vi "One Shot Single Tone - no AO.vi"() -> ()   [LabVIEW 2021]
doc: "This VI generates and acquires data for a single-shot acquisition and performs gain and total harmonic distortion (THD) measurements on the acquired response channel. You can specify the initial settling time of the device under test, the integration time to use for the measurement, and the frequency range of interest. \n\nThe graphical outputs display the time record of the acquired response and the magnitude spectrum versus frequency, respectively. You can also investigate the contribution of each harmonic component to the THD.\n\nRequirements:\nLabVIEW Full Development System\nSound and Vibration Toolkit\n\nInstructions:\n1. Connect DUT to DAQmx hardware.\n2. Specify connected output channel and input channel (response).\n3. Use SVL Measure Propagation Delay (DAQmx) VI to measure device propagation delay [samples].\n4. Run the VI.\n\nDetails:\nThis VI measures the gain and total harmonic distortion (THD) of a device under test (DUT). It generates a single-tone stimulus to excite the DUT. The gain is the ratio of output to input amplitudes. THD quantifies the level of non-linear harmonics produced from excitation at a single frequency. THD is defined as the ratio of the RMS sum of the harmonic levels to the level of the fundamental frequency. \n\nRefer to the wiring diagram to physically connect the DSA or DAQ device to the DUT. This example uses one analog input channel and one analog output channel. \n\nThe wiring diagram assumes that you use the default channel settings. If you change the channel settings in the VI front panel you should adjust the physical connections appropriately.\n\nNI strongly recommends that you take precautions to limit the effects of out-of-band aliasing in your frequency domain measurements. DSA devices use transparent digital and analog hardware filtering to eliminate aliased input and output frequencies. Multifunction DAQ devices are more susceptible to the effects of aliased frequencies. If you are using a non-DSA measurement device, we recommend addressing potential aliasing through high sampling rates, built-in analog filters on S Series devices, and/or external analog filters."
uses:
  <vilib>/addons/_XControls/Spectrum with Cursors/Spectrum with Cursors.xctl
  <vilib>/addons/_NISVFA/_Shared subVIs/Data Objects/Data/Data.lvclass
  <vilib>/addons/_XControls/Waveforms with Cursors/Waveforms with Cursors.xctl
  <vilib>/addons/_NISVFA/_Generation/Signal Generation/SV Signal/sv_System Timing Model.ctl
  Program Files/National Instruments/LabVIEW 2021/examples/Sound and Vibration/Audio Measurements/subVIs/sv_AO Channel Configuration.ctl
  Program Files/National Instruments/LabVIEW 2021/examples/Sound and Vibration/Audio Measurements/subVIs/sv_AI Channel Configuration.ctl
  <vilib>/addons/_NISVFA/_Generation/Signal Generation/SV Signal/SV Signal.lvclass/SV Signal.ctl
  <vilib>/addons/_NISVFA/_Shared subVIs/Controls/svc_Window.ctl
  <vilib>/addons/_NISVFA/_Shared subVIs/Data Objects/Data/Data.lvclass/Data.ctl
  <vilib>/addons/_NISVFA/_Generation/Signal Generation/SV Signal/Write Synchronization Pulse Parameters.vi
  <vilib>/addons/_NISVFA/_Generation/Signal Generation/SV Signal/Write Ramp-Up.vi
  <vilib>/addons/_NISVFA/_Generation/Signal Generation/SV Signal/Write Ramp-Down.vi
  <vilib>/addons/_NISVFA/_Generation/Signal Generation/SV Signal/Write Profile.vi
  <vilib>/Analysis/1siggen.llb/Ramp Pattern by Samples.vi
  <vilib>/addons/_NISVFA/_Shared subVIs/Common/SVL Set dB Reference (1 Ch).vi
  <vilib>/addons/Sound and Vibration/svt_Level/SVL AC & DC Level (Time) (1 Ch).vi
  <vilib>/addons/_NISVFA/_Shared subVIs/Data Objects/Y (Complex) (DBL)/SV Convert Complex Spectrum to Data Object.vi
  <vilib>/addons/Sound and Vibration/svt_Single Tone Measurements/SVT Spurious Free Dynamic Range (Frequency) (1 Ch).vi
  <vilib>/DAQmx/read.llb/DAQmx Read.vi
  <vilib>/DAQmx/read.llb/DAQmx Read (Analog 1D Wfm NChan NSamp).vi
  Program Files/National Instruments/LabVIEW 2021/examples/Sound and Vibration/Audio Measurements/subVIs/sv_Modify Channel Names.vi
  Program Files/National Instruments/LabVIEW 2021/examples/Sound and Vibration/Audio Measurements/subVIs/sv_Synchronize DSA AI and AO Tasks.vi
  <vilib>/DAQmx/write.llb/DAQmx Write.vi
  <vilib>/DAQmx/write.llb/DAQmx Write (Analog Wfm 1Chan NSamp).vi
  Program Files/National Instruments/LabVIEW 2021/examples/Sound and Vibration/Audio Measurements/subVIs/sv_Synchronization Gatekeeper.vi
  Program Files/National Instruments/LabVIEW 2021/examples/Sound and Vibration/Audio Measurements/subVIs/sv_Synchronize Acquisition and Generation.vi
  Program Files/National Instruments/LabVIEW 2021/examples/Sound and Vibration/Audio Measurements/subVIs/sv_Prepare Acquired Waveforms for Parsing.vi
  <vilib>/addons/_NISVFA/_Shared subVIs/Common/SVL Set dB Reference (variant).vi
  <vilib>/addons/_NISVFA/_Shared subVIs/Common/svc_Get SV Channel Info.vi
  <vilib>/Analysis/baseanly.llb/Mean.vi
  <vilib>/Analysis/baseanly.llb/Mean (DBL).vi
  <vilib>/addons/_NISVFA/_Shared subVIs/Windowing/svfa_Scaled Time Domain Window (Array).vi
  <vilib>/addons/_NISVFA/_Shared subVIs/Common/sv_Get NI Property Name String.vi
  <vilib>/addons/_NISVFA/_Shared subVIs/Data Objects/Data/Write Data Attributes.vi
  <vilib>/addons/_NISVFA/_Spectrum Processing/SVFA Get Spectrum Subset.vi
  <vilib>/addons/_NISVFA/_Spectrum Processing/SVFA Get Spectrum Subset (Complex) (1 Ch).vi
  <vilib>/addons/_NISVFA/_Shared subVIs/Common/svc_Window Parameters.vi
  <vilib>/addons/_NISVFA/_Shared subVIs/Common/svc_Extract Single Tone Information (complex).vi
  <vilib>/addons/_NISVFA/_Shared subVIs/Common/svc_Check Frequency Range in Spectrum.vi
  <vilib>/addons/_NISVFA/_Spectrum Processing/SVFA Unit Conversion.vi
  <vilib>/addons/_NISVFA/_Spectrum Processing/SVFA Unit Conversion (Complex) (1 Ch).vi
  <vilib>/addons/_NISVFA/_Spectrum Processing/SVFA Spectrum Peak Search.vi
  <vilib>/addons/_NISVFA/_Spectrum Processing/SVFA Spectrum Peak Search (1 Ch).vi
  <vilib>/addons/_NISVFA/_Shared subVIs/Common/svc_Spectrum Units.vi
  Program Files/National Instruments/LabVIEW 2021/examples/Sound and Vibration/Audio Measurements/subVIs/sv_Synchronization Keymaster.vi
  <vilib>/Utility/error.llb/Clear Errors.vi
  Program Files/National Instruments/LabVIEW 2021/examples/Sound and Vibration/Audio Measurements/subVIs/sv_Get Reference Clock.vi
  Program Files/National Instruments/LabVIEW 2021/examples/Sound and Vibration/Audio Measurements/subVIs/sv_Synchronization Keymaster_GO.vi
  <extravilib>/ChannelInstances/Tag-c(ref(UserDefinedRefnumTag),t'Rendezvous RefNum')/Read.vi
  Program Files/National Instruments/LabVIEW 2021/examples/Sound and Vibration/Audio Measurements/subVIs/sv_Timing for Stimulus Response Tasks.vi
  <vilib>/addons/_NISVFA/_Generation/Signal Generation/SV Signal/Read Total Samples.vi
  <vilib>/addons/_NISVFA/_Generation/Signal Generation/SV Signal/Write Leading Synchronization Pulse Enable.vi
  Program Files/National Instruments/LabVIEW 2021/examples/Sound and Vibration/Audio Measurements/subVIs/sv_Align Waveforms by Leading Sync Pulse.vi
  <vilib>/addons/_NISVFA/_Generation/Signal Generation/SV Signal/Read Synchronization Pulse Waveform.vi
  <vilib>/addons/_NISVFA/_Shared subVIs/Common/svc_Check for Waveform Parameter Continuity (N Ch).vi
  Program Files/National Instruments/LabVIEW 2021/examples/Sound and Vibration/Audio Measurements/subVIs/sv_Append Virtual Reference.vi
  <vilib>/addons/_NISVFA/_Shared subVIs/Common/svc_Unit Label to Engineering Units.vi
  <vilib>/addons/_NISVFA/_Shared subVIs/Common/svc_Engineering Units to Unit Label.vi
  <vilib>/addons/_NISVFA/_Spectrum Processing/subVIs/svfa_Spectrum Info Window to windowTd Type Def.vi
  <vilib>/Analysis/4window.llb/Force Window.vi
  <vilib>/Analysis/4window.llb/Force Window (DBL).vi
  <vilib>/Analysis/4window.llb/Exponential Window.vi
  <vilib>/Analysis/4window.llb/Exponential Window (DBL).vi
  <vilib>/addons/_NISVFA/_Shared subVIs/Data Objects/Data/Read Data Attributes.vi
  <vilib>/addons/_NISVFA/_Shared subVIs/Common/svc_Build Unit Label for Frequency Range.vi
  <vilib>/addons/_NISVFA/_Spectrum Processing/SVFA Get Tone Amplitude and Phase (1 Ch).vi
  <vilib>/addons/_NISVFA/_Spectrum Processing/subVIs/svfa_Compute Complex Spectrum for Export.vi
  <vilib>/addons/_NISVFA/_Shared subVIs/Common/svc_Check Frequency Range in Bandwidth.vi
  <vilib>/addons/_NISVFA/_Shared subVIs/Common/svc_Convert Start and Stop to Start Index and Length.vi
  <vilib>/addons/_NISVFA/_Shared subVIs/Common/svc_Log View for Spectrum (1Ch).vi
  <vilib>/addons/_NISVFA/_Spectrum Processing/SVFA Unit Conversion (1 Ch).vi
  <vilib>/addons/_NISVFA/_Shared subVIs/Common/svc_Complex Datatype Defaults.vi
  <vilib>/addons/_NISVFA/_Spectrum Processing/subVIs/svfa_Spectrum Peak Search.vi
  <vilib>/addons/_NISVFA/_Shared subVIs/Common/svc_Format Value (DBL).vi
  <vilib>/addons/_NISVFA/_Shared subVIs/Common/svc_Get Weighting Enum and Labels.vi
  <vilib>/addons/_NISVFA/_Shared subVIs/Common/svc_Surround NonAlpha String with Parentheses.vi
  <vilib>/dlg_ctls.llb/Space Constant.vi
  <extravilib>/ChannelInstances/Tag-c(ref(UserDefinedRefnumTag),t'Rendezvous RefNum')/Write.vi
  <extravilib>/ChannelInstances/Tag-c(ref(UserDefinedRefnumTag),t'Rendezvous RefNum')/Read With Abort.vi
  <vilib>/addons/_NISVFA/_Generation/Signal Generation/SV Signal/Calculate Number of Remaining Samples.vi
  Program Files/National Instruments/LabVIEW 2021/examples/Sound and Vibration/Audio Measurements/subVIs/sv_Measure Delay for Active and Idle Channels.vi
  <vilib>/addons/_NISVFA/_Generation/Signal Generation/SV Signal/Read Leading Synchronization Pulse Enable.vi
  <vilib>/addons/_NISVFA/_Generation/Signal Generation/SV Signal/Read Trailing Synchronization Pulse Enable.vi
  <vilib>/addons/_NISVFA/_Shared subVIs/Common/svc_Check for Waveform Parameter Continuity (no state).vi
  <vilib>/addons/_NISVFA/_Spectrum Processing/subVIs/svfa_Window Frequency Response.vi
  <vilib>/addons/_NISVFA/_Spectrum Processing/subVIs/svfa_Window Frequency Response (double array).vi
  <vilib>/Analysis/baseanly.llb/Dot Product.vi
  <vilib>/Analysis/baseanly.llb/Complex Dot Product.vi
  <vilib>/addons/_NISVFA/_Shared subVIs/Common/svc_Unwrap Phase.vi
  <vilib>/addons/_NISVFA/_Shared subVIs/Common/svc_Convert Spectrum Array to dB.vi
  <vilib>/addons/_NISVFA/_Spectrum Processing/subVIs/svfa_Conversion Utility (spectrum info).vi
  <vilib>/addons/_NISVFA/_Spectrum Processing/subVIs/svfa_Peak Rough Search Indices.vi
  <vilib>/addons/_NISVFA/_Shared subVIs/Common/svc_Unit Label Lexical Class.vi
  <extravilib>/ChannelInstances/Tag-c(ref(UserDefinedRefnumTag),t'Rendezvous RefNum')/Write With Abort.vi
  <vilib>/addons/Sound and Vibration/svt_Calibration/SV Measure Delay and Polarity and Coherence (Nx1).vi
  Program Files/National Instruments/LabVIEW 2021/examples/Sound and Vibration/Audio Measurements/subVIs/sv_Assign Delay to Idle Channels.vi
  <vilib>/addons/_NISVFA/_Spectrum Processing/subVIs/svfa_Rect Window Frequency Response.vi
  <vilib>/addons/_NISVFA/_Spectrum Processing/subVIs/svfa_Cosine Window Coefficients.vi
  <vilib>/addons/_NISVFA/_Spectrum Processing/subVIs/svfa_Peak to RMS to Peak2Peak.vi
  <vilib>/addons/_NISVFA/_Spectrum Processing/subVIs/svfa_Mag to Mag2.vi
  <vilib>/addons/_NISVFA/_Spectrum Processing/subVIs/svfa_Linear to dB.vi
  <vilib>/addons/_NISVFA/_Spectrum Processing/subVIs/svfa_dBrefA to dBrefB.vi
  <vilib>/addons/_NISVFA/_Spectrum Processing/subVIs/svfa_Spectrum to Spectral Density.vi
  <vilib>/addons/Sound and Vibration/svt_Calibration/SV Measure Delay and Polarity and Coherence.vi
  <vilib>/Analysis/_algsub.llb/Vector Norm.vi
  <vilib>/Analysis/_algsub.llb/Real Vector Norm.vi
  <vilib>/addons/_NISVFA/_Shared subVIs/Common/SV Get Data Subset.vi
  <vilib>/addons/_NISVFA/_Shared subVIs/Common/svc_Get Array Subset (Index).vi
  <vilib>/addons/_NISVFA/_Shared subVIs/Common/svc_Coerce Index and Length.vi
  <vilib>/addons/_NISVFA/_Shared subVIs/Common/svc_Conditional Merge Error.vi
  <vilib>/addons/_NISVFA/_Generation/Signal Generation/SV Sinusoid/SV Sinusoid.lvclass
  C:/Program Files/National Instruments/LabVIEW 2021/vi.lib/addons/_NISVFA/_Generation/Signal Generation/SV Signal/SV Signal.lvclass
  C:/Program Files/National Instruments/LabVIEW 2021/vi.lib/addons/_NISVFA/_Generation/Signal Generation/SV Function/SV Function.lvclass
  <vilib>/addons/_NISVFA/_Shared subVIs/Data Objects/Y (Complex) (DBL)/Y (Complex) (1 Ch).lvclass
  C:/Program Files/National Instruments/LabVIEW 2021/vi.lib/addons/_NISVFA/_Shared subVIs/Data Objects/Data/Data.lvclass
  <vilib>/addons/_NISVFA/_Generation/Signal Generation/SV Sinusoid/Configure Sine.vi
  <vilib>/addons/_NISVFA/_Generation/Signal Generation/SV Signal/Write System Timing Model.vi
  <vilib>/addons/_NISVFA/_Generation/Signal Generation/SV Signal/Write Transition Profile.vi
  <vilib>/addons/_NISVFA/_Generation/Signal Generation/SV Signal/Write Measurement Duration.vi
  <vilib>/addons/_NISVFA/_Generation/Signal Generation/SV Function/Write Measurement Cycles.vi
  <vilib>/addons/_NISVFA/_Generation/Signal Generation/SV Signal/Write Pre-Measurement Settling Duration.vi
  <vilib>/addons/_NISVFA/_Generation/Signal Generation/SV Function/Write Pre-Measurement Settling Cycles.vi
  <extravilib>/ChannelInstances/Tag-c(ref(UserDefinedRefnumTag),t'Rendezvous RefNum')/Instantiate.vi
  Program Files/National Instruments/LabVIEW 2021/examples/Sound and Vibration/Audio Measurements/subVIs/sv_Configure AI Task.vi
  Program Files/National Instruments/LabVIEW 2021/examples/Sound and Vibration/Audio Measurements/subVIs/sv_Configure AO Task.vi
  <vilib>/addons/_NISVFA/_Generation/Signal Generation/SV Signal/Read Sample Rate.vi
  <vilib>/addons/_NISVFA/_Generation/Signal Generation/SV Signal/Read Generation State.vi
  <vilib>/addons/_NISVFA/_Generation/Signal Generation/SV Signal/Read System Timing Model.vi
  <vilib>/DAQmx/configure/timing.llb/DAQmx Timing.vi
  <vilib>/DAQmx/configure/timing.llb/DAQmx Timing (Sample Clock).vi
  <vilib>/addons/_NISVFA/_Generation/Signal Generation/SV Signal/Write Sample Rate.vi
  <extravilib>/ChannelInstances/Tag-c(ref(UserDefinedRefnumTag),t'Rendezvous RefNum')/EndpointRead.vi
  <vilib>/Utility/rendezvs.llb/Wait at Rendezvous.vi
  <vilib>/DAQmx/configure/task.llb/DAQmx Stop Task.vi
  Program Files/National Instruments/LabVIEW 2021/examples/Sound and Vibration/Audio Measurements/subVIs/sv_Get Bus Type and Product Type.vi
  <vilib>/DAQmx/configure/task.llb/DAQmx Control Task.vi
  <vilib>/Utility/rendezvs.llb/Create Rendezvous.vi
  <extravilib>/ChannelInstances/Tag-c(ref(UserDefinedRefnumTag),t'Rendezvous RefNum')/Endpoint.vi
  <vilib>/addons/Sound and Vibration/svt_DAQmx/subVIs/svl_Get Terminal Name with Device Prefix.vi
  <vilib>/DAQmx/configure/trigger.llb/DAQmx Trigger.vi
  <vilib>/DAQmx/configure/trigger.llb/DAQmx Start Trigger (Digital Edge).vi
  <vilib>/DAQmx/configure/task.llb/DAQmx Start Task.vi
  <vilib>/Utility/rendezvs.llb/Destroy Rendezvous.vi
  <vilib>/DAQmx/miscellaneous.llb/DAQmx Fill In Error Info.vi
  <vilib>/DAQmx/configure/task.llb/DAQmx Clear Task.vi
  <vilib>/addons/_NISVFA/_Shared subVIs/Data Objects/Waveforms (DBL)/Write to Buffer.vi
  <vilib>/addons/_NISVFA/_Shared subVIs/Data Objects/Waveforms (DBL)/Read from Buffer.vi
  <vilib>/addons/_NISVFA/_Shared subVIs/Data Objects/Waveforms (DBL)/SV Read Newest Data.vi
  <vilib>/measure/maresamp.llb/Resample Waveforms (single shot).vi
  <vilib>/measure/maresamp.llb/Resample Waveform (single shot).vi
  <vilib>/addons/_NISVFA/_Shared subVIs/Common/svc_Check dt for Equal Sample Rates.vi
  <vilib>/Waveform/TSOps.llb/Timestamp Subtract.vi
  <vilib>/Analysis/2dsp.llb/CrossCorrelation.vi
  <vilib>/Analysis/2dsp.llb/1D Cross Correlation (DBL).vi
  <vilib>/addons/_NISVFA/_Shared subVIs/Common/svc_Fit Quadratic to Max Three Points in Array.vi
  <vilib>/Utility/error.llb/Error Cluster From Error Code.vi
  <vilib>/addons/_NISVFA/_Shared subVIs/Common/svc_Caller VI Returned in Error Source.vi
  <vilib>/addons/_NISVFA/_Shared subVIs/Common/SV Remove Delays (1,N) from Waveforms (N Ch) (DBL).vi
  <vilib>/addons/_NISVFA/_Shared subVIs/Common/SV Remove Delays from Waveforms.vi
  <vilib>/addons/_NISVFA/_Shared subVIs/Data Objects/Waveforms (DBL)/SV Read Next Measurement Data.vi
  <vilib>/addons/_NISVFA/_Shared subVIs/Common/svc_Get Window Info.vi
  <vilib>/Analysis/0measdsp.llb/Scaled Time Domain Window.vi
  <vilib>/Analysis/0measdsp.llb/Scaled Time Domain Window (DBL).vi
  <vilib>/Analysis/baseanly.llb/Std Deviation and Variance.vi
  <vilib>/addons/Sound and Vibration/svt_Single Tone Measurements/SVT Gain (Time) (1 Ch).vi
  <vilib>/addons/_NISVFA/_Shared subVIs/Data Objects/Y (Complex) (DBL)/Write Y.vi
  <vilib>/addons/_NISVFA/_Shared subVIs/Spectrum Info/sv_Convert Spectrum Info to Variant Attributes.vi
  <vilib>/addons/_NISVFA/_Spectrum Processing/SVFA Extract Multiple Tone Information (Complex) (1 Ch).vi
  <vilib>/addons/Sound and Vibration/svt_Distortion/SVT THD and Harmonic Components (Frequency) (1 Ch).vi
  <vilib>/addons/Sound and Vibration/svt_Distortion/SVT SNR without Harmonics (Frequency) (1 Ch).vi
  <vilib>/addons/Sound and Vibration/svt_Single Tone Measurements/SVT Dynamic Range (Frequency) (1 Ch).vi
  <vilib>/addons/Sound and Vibration/svt_Distortion/subVIs/sv_Check Data Valid (Audio) (1 Ch).vi
  <vilib>/addons/_NISVFA/_Shared subVIs/Common/svc_Convert Frequency to Frequency String.vi
  <vilib>/Analysis/4window.llb/window parameters.vi
  <vilib>/Analysis/4window.llb/Window Properties.vi
  <vilib>/Analysis/4window.llb/Window Properties by Name.vi
  <vilib>/addons/_NISVFA/_Spectrum Processing/subVIs/svfa_Spectrum Peak Tone Search and Estimation (complex).vi
  <vilib>/measure/masignal.llb/Tones and Noise Waveform.vi
  <vilib>/addons/_NISVFA/_Shared subVIs/Common/svc_FFT with Window.vi
  <vilib>/Analysis/1siggen.llb/Square Wave.vi
  <vilib>/addons/_NISVFA/_Spectrum Processing/subVIs/svfa_Three Finger Peak Search.vi
  <vilib>/addons/Sound and Vibration/svt_Distortion/subVIs/sv_Peak View Amplitude (1 Ch).vi
  <vilib>/addons/_NISVFA/_Generation/Signal Generation/SV Signal/SV Signal.lvclass
  <vilib>/addons/Sound and Vibration/svt_Single Tone Measurements/SoundVib_SingleTone.lvlib
  <vilib>/addons/Sound and Vibration/svt_Distortion/SoundVib_Distortion.lvlib
  <vilib>/Analysis/NI_AALBase.lvlib
  Program Files/National Instruments/LabVIEW 2021/examples/Sound and Vibration/SoundVib_Audio Examples.lvlib
panel:
  out "Waveforms with Cursors":waveform(dbl)[](xcontrol)
  out "Spectrum with Cursors":refnum<class "Data.lvclass">(xcontrol)
  in  "Settings":T1(tab)
  in  "AO range":dbl=3.5 format="±  %.3g"
  in  "input channel":tag="Dev1/ai0"
  in  "output channel":tag="Dev1/ao0"
  in  "AI range":dbl=3.0 format="±  %.3g"
  in  "amplitude units":enum16{"V", "dB FS"}(ring)
  in  "full scale (V pk)":dbl=3.16 format="%.3p"
  in  "amplitude":dbl=1.0 format="%.3g"
  in  "frequency (Hz)":dbl=1000.0 min=20.0 max=100000.0 step=1.0 format="%.2f"
  in  "frequency range":T2={"band start (Hz)"=20.0, "band stop (Hz)"=20000.0} {"band stop (Hz)" format="%.2f"; "band start (Hz)" format="%.2f"}
  in  "Rub & Buzz maximum harmonic":i32=20 min=-1 max=1000
  in  "measurement cycles":dbl=20.0 min=1.0
  in  "measurement duration (s)":dbl=0.05 min=0.0 format="%.2p"
  in  "THD maximum harmonic":i32=9 min=-1 max=1000
  in  "settle cycles":dbl=10.0 min=0.0
  in  "settle time (s)":dbl=0.01 min=0.0 format="%.2p"
  in  "ramp down (s)":dbl=0.01 min=0.0 format="%.2p"
  in  "ramp up (s)":dbl=0.02 min=0.0 format="%.2p"
  out "Rub & Buzz distortion (%)":dbl format="%_4g"
  out "THD (dB)":dbl format="%.1f"
  out "gain (dB)":dbl format="%.3f"
  out "fundamental amplitude (V)":dbl format="%_6g"
  out "fundamental frequency (Hz)":dbl format="%_6g"
  out "2X amplitude (V)":dbl format="%_4g"
  out "3X amplitude (V)":dbl format="%_4g"
  out "4X amplitude (V)":dbl format="%_4g"
  out "5X amplitude (V)":dbl format="%_4g"
  out "6X amplitude (V)":dbl format="%_4g"
  out "7X amplitude (V)":dbl format="%_4g"
  out "SNR (dB)":dbl format="%.1f"
  out "THD (%)":dbl format="%_4f"
  out "THD+N (dB)":dbl format="%.1f"
  out "Dynamic Range (dB FS)":dbl format="%.1f"
  out "SFDR (dB)":dbl format="%.1f"
  # "Results"
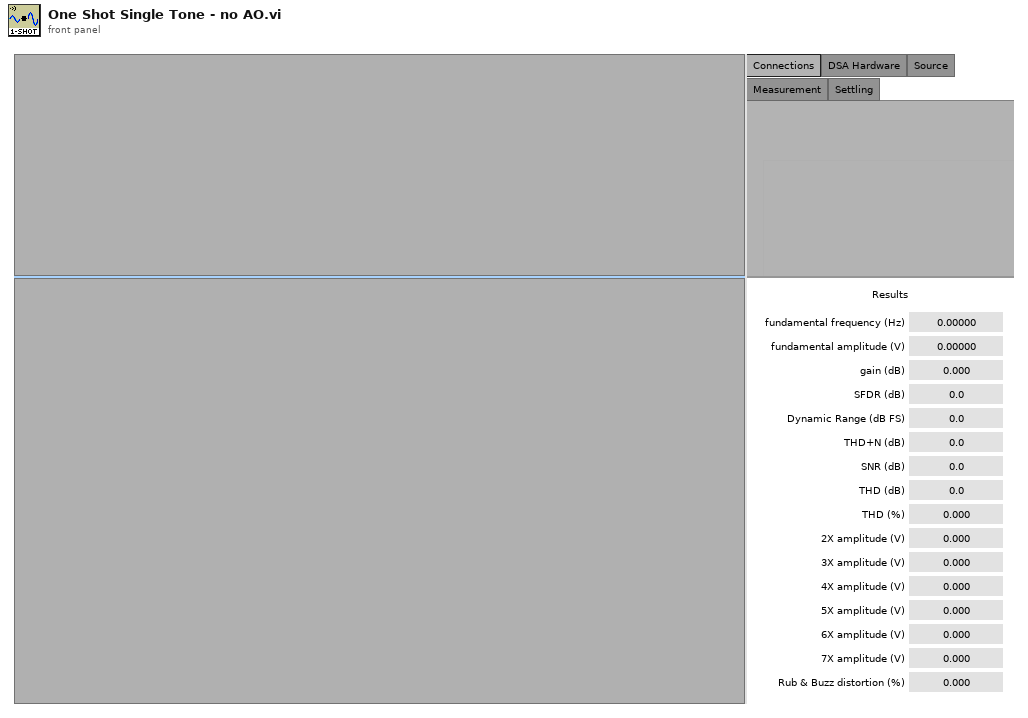
[diagram p1: front panel]
types:
  T1 = enum32{"Connections", "DSA Hardware", "Source", "Measurement", "Settling"}
  T2 = cluster{"band start (Hz)":dbl, "band stop (Hz)":dbl}
  T3 = typedef "SoundVib_Audio Examples.lvlib/sv_AI Channel Configuration.ctl" = cluster{"DAQmx Channel":tag, "Channel Type":u16, "Max":dbl, "Sensitivity":dbl, "Coupling":enum16{"AC", "DC"}, "excitation":enum16{"Off", "Min", "Max"}, "input terminal configuration":i32}
  T4 = typedef "SoundVib_Audio Examples.lvlib/sv_AO Channel Configuration.ctl" = cluster{"DAQmx Channel":tag, "Max":dbl, "output terminal configuration":i32}
  T5 = cluster{"enable leading":bool, "enable trailing":bool, "duration [s]":dbl, "type":enum16{"Noise", "MLS", "Chirp", "Monopulse", "Custom"}, "level":dbl}
  T6 = cluster{"SNR units":enum16{"dB", "linear ratio", "%"}, "detected fundamental amplitude units":enum16{"EU rms", "EU peak", "EU peak-peak"}}
  T7 = cluster{"THD units":enum16{"dB", "linear ratio", "%"}, "harmonic component amplitude units":enum16{"EU rms", "EU peak", "EU peak-peak", "dB ref fund"}, "detected fundamental amplitude units":enum16{"EU rms", "EU peak", "EU peak-peak"}}
  T8 = cluster{"gain units":enum16{"dB", "linear ratio"}, "detected fundamental amplitude units":enum16{"EU rms", "EU peak", "EU peak-peak"}}
  T9 = typedef "SV Signal.lvclass/sv_System Timing Model.ctl" = i64
  T10 = typedef "svc_Window.ctl" = u32
  T11 = typedef "svc_Spectrum Info.ctl" = cluster{"channel name":string, "description":string, "x-axis units":T12, "spectral info":cluster{"spectrum type":T13, "linear/dB":enum16{"linear", "dB"}, "window":u16, "window size":i32, "FFT size":i32}, "engineering units":T14, "custom label":string, "dB reference [EU]":dbl, "peak units":enum16{"rms", "peak", "peak-peak"}, "weighting filter":T15, "spectral density?":bool, "unit label":string, "spectrum skewed?":bool, "complimentary spectrum units":T16}
  T12 = typedef "svc_X-Axis Units.ctl" = u16
  T13 = typedef "svc_Spectrum Type.ctl" = enum16{"FFT Spectrum [complex]", "Amplitude [Magnitude]", "Power [Magnitude^2]", "Cross Spectrum [complex]", "Frequency Response [Complex]"}
  T14 = typedef "svc_Engineering Units Text Ring.ctl" = u16
  T15 = typedef "svc_Weighting Filter Text Ring.ctl" = u16
  T16 = typedef "svc_Complimentary Spectrum Units.ctl" = enum16{"none", "radians", "degrees", "cycles", "imaginary"}
  T17 = cluster{"complex spectrum response":cluster{"f0":dbl, "df":dbl, "complex spectrum":cdb[]}, "spectrum info":T11}
  T18 = cluster{"frequency [Hz]":dbl, "amplitude [EU pk]":dbl, "phase (deg)":dbl}[]
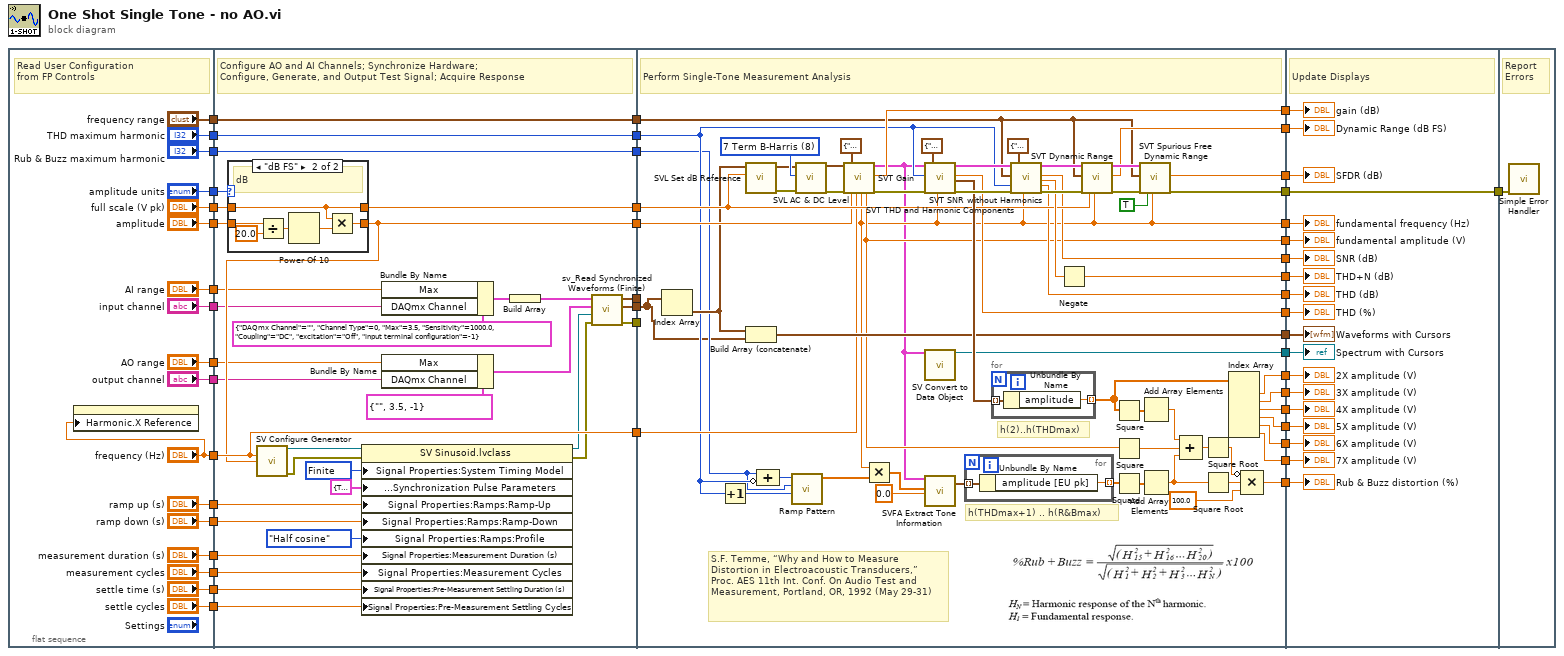
[diagram p0: block diagram]
diagram:
  n1 = flat-sequence {
    tunnel: ["frequency range"] -> w46
    tunnel: ["THD maximum harmonic"] -> w45
    tunnel: ["frequency (Hz)"] -> w44
    tunnel: ["measurement duration (s)"] -> w43
    tunnel: ["measurement cycles"] -> w42
    tunnel: ["settle time (s)"] -> w41
    tunnel: ["settle cycles"] -> w40
    tunnel: ["output channel"] -> w39
    tunnel: ["input channel"] -> w38
    tunnel: ["AI range"] -> w37
    tunnel: ["AO range"] -> w36
    tunnel: ["full scale (V pk)"] -> w35
    tunnel: ["ramp down (s)"] -> w34
    tunnel: ["ramp up (s)"] -> w33
    tunnel: ["amplitude"] -> w32
    tunnel: ["amplitude units"] -> w31
    tunnel: ["Rub & Buzz maximum harmonic"] -> w30
    tunnel: w46 -> [w97]
    tunnel: w45 -> [w87]
    tunnel: w44 -> [w81]
    tunnel: w43 -> [w92]
    tunnel: w42 -> [w91]
    tunnel: w41 -> [w90]
    tunnel: w40 -> [w89]
    tunnel: w39 -> [w64]
    tunnel: w38 -> [w66]
    tunnel: w37 -> [w67]
    tunnel: w36 -> [w65]
    tunnel: w35 -> [w94]
    tunnel: w34 -> [w82]
    tunnel: w33 -> [w83]
    tunnel: w32 -> [w93]
    tunnel: w31 -> [w86]
    tunnel: w30 -> [w85]
    tunnel: [w97] -> w9
    tunnel: [w88] -> w8
    tunnel: [w87] -> w7
    tunnel: [w76] -> w6
    tunnel: [w81] -> w5
    tunnel: [w85] -> w4
    tunnel: [w79] -> w3
    tunnel: [w78] -> w2
    tunnel: [w77] -> w1
    tunnel: [w133] -> w29
    tunnel: [w132] -> w28
    tunnel: [w131] -> w27
    tunnel: [w130] -> w26
    tunnel: [w129] -> w25
    tunnel: [w128] -> w24
    tunnel: [w127] -> w23
    tunnel: [w107] -> w22
    tunnel: [w126] -> w21
    tunnel: [w125] -> w20
    tunnel: [w124] -> w19
    tunnel: [w123] -> w18
    tunnel: [w122] -> w17
    tunnel: [w121] -> w16
    tunnel: [w120] -> w15
    tunnel: [w119] -> w14
    tunnel: [w118] -> w13
    tunnel: [w117] -> w12
    tunnel: [w116] -> w11
    tunnel: w9 -> [w109]
    tunnel: w8 -> [w136]
    tunnel: w7 -> [w112]
    tunnel: w6 -> [w135]
    tunnel: w5 -> [w115]
    tunnel: w4 -> [w108]
    tunnel: w3 -> [_]
    tunnel: w2 -> [w106]
    tunnel: w1 -> [_]
    tunnel: w29 -> [w191]
    tunnel: w28 -> [w190]
    tunnel: w27 -> [w189]
    tunnel: w26 -> [w188]
    tunnel: w25 -> [w175]
    tunnel: w24 -> [w187]
    tunnel: w23 -> [w186]
    tunnel: w22 -> [w173]
    tunnel: w21 -> [w185]
    tunnel: w20 -> [w184]
    tunnel: w19 -> [w183]
    tunnel: w18 -> [w182]
    tunnel: w17 -> [w181]
    tunnel: w16 -> [w180]
    tunnel: w15 -> [w179]
    tunnel: w14 -> [w178]
    tunnel: w13 -> [w177]
    tunnel: w12 -> [w176]
    tunnel: w11 -> [w174]
    tunnel: [w175] -> w10
    tunnel: w10 -> [w192]
    frame #0 {
      # "Read User Configuration\nfrom FP Controls"
      n2 = property on="Spectrum with Cursors" class="Spectrum with Cursors (strict)"("Harmonic.X Reference"="frequency (Hz)") -> ()  [unwired: 2 in, 2 out]
    }
    frame #1 {
      w96 = T9 10178 items=["Finite"=10178, "-"=-1, "Continuous"=10123, "-"=-2, "Settled"=110123, "Averaged"=210123, "Discrete Sweep"=310123, "Continuous Sweep"=410123] ("System Timing Model")
      # "Configure AO and AI Channels; Synchronize Hardware; \nConfigure, Generate, and Output Test Signal; Acquire Response"
      n3 = case shown="\"dB FS\"" w86 {
        tunnel: [w99 w101] -> w76
        tunnel: w93 -> [w99 w105]
        tunnel: w94 -> [w98 w100]
        tunnel: [w98 w100] -> w88
        frame Default {
          # "V"
        }
        frame "dB FS" {
          # "dB"
          n4 = Divide(x=w105, y=20.0) -> (x/y=w103:dbl)
          n5 = Power Of 10(x=w103) -> (10^x=w102:dbl)
          n6 = Multiply(x=w100, y=w102) -> (x*y=w101:dbl)
        }
      }
      n7 = call-poly <vilib>:"SV Configure Generator.vi"("frequency (Hz)"=w81, "amplitude"=w76) -> ("signal configuration"=w95:refnum<class "SV Sinusoid.lvclass">, "error out"=w73:errorcluster)  [unwired: 12 in]
      n8 = property class="SV Sinusoid.lvclass"(reference=w95, error in=w73, "Signal Properties:System Timing Model"=w96, "Signal Properties:Synchronization Pulses:Synchronization Pulse Parameters"=T5 {"enable leading"=TRUE, "enable trailing"=FALSE, "duration [s]"=0.005, "type"=enum."Noise", "level"=0.5} ("Synchronization Pulses:All Elements"), "Signal Properties:Ramps:Ramp-Up"=w83, "Signal Properties:Ramps:Ramp-Down"=w82, "Signal Properties:Ramps:Profile"=enum16{"Linear", "Half cosine"}."Half cosine" ("Ramp Parameters:Profile"), "Signal Properties:Measurement Duration (s)"=w92, "Signal Properties:Measurement Cycles"=w91, "Signal Properties:Pre-Measurement Settling Duration (s)"=w90, "Signal Properties:Pre-Measurement Settling Cycles"=w89) -> (reference out=w74:refnum<class "SV Sinusoid.lvclass">, error out=w75:errorcluster)
      n9 = Bundle By Name(cluster=T3 {"DAQmx Channel"="", "Channel Type"=0, "Max"=3.5, "Sensitivity"=1000.0, "Coupling"=enum."DC", "excitation"=enum."Off", "input terminal configuration"=-1} ("Channel Information"), "Max"=w67, "DAQmx Channel"=w66) -> (w70:T3)
      n10 = Bundle By Name(cluster=T4 {"DAQmx Channel"="", "Max"=3.5, "output terminal configuration"=-1} ("analog output channel"), "Max"=w65, "DAQmx Channel"=w64) -> (w68:T4)
      n11 = Build Array(w70) -> (w69:T3[])
      n12 = call "sv_Read Synchronized Waveforms (Finite).vi"("error in (no error)"=w75, "signal configuration in"=w74, "analog output channel"=w68, "analog input channels"=w69) -> ("error out"=w77:errorcluster, "full waveforms"=w78:waveform(dbl)[], "waveforms to measure"=w79:waveform(dbl)[])  [unwired: 3 in, 2 out]
    }
    frame #2 {
      w167 = T10 8 items=["None"=0, "Hanning"=1, "Hamming"=2, "Blackman-Harris"=3, "Exact Blackman"=4, "Blackman"=5, "Flat Top"=6, "4 Term B-Harris "=7, "7 Term B-Harris"=8, "Low Sidelobe"=9, "Force"=64, "Exponential"=65, "Blackman Nuttall"=11, "Triangle"=30, "Bartlett-Hanning"=31, "Bohman"=32, "Parzen"=33, "Welch"=34, "Kaiser"=60, "Dolph-Chebyshev"=61, "Gaussian"=62] ("window")
      # "S.F. Temme, “Why and How to Measure Distortion in Electroacoustic Transducers,” \nProc. AES 11th Int. Conf. On Audio Test and Measurement, Portland, OR, 1992 (May 29-31)"
      # "h(THDmax+1) .. h(R&Bmax)"
      # "h(2)..h(THDmax)"
      # "Perform Single-Tone Measurement Analysis"
      n13 = Index Array(array=w106) -> (element=w134:waveform(dbl))  [unwired: 1 in]
      n14 = Increment(x=w112) -> (x+1=w113:i32)
      n15 = call-poly <vilib>:"SVL Set dB Reference.vi"("dB reference [EU]"=w136, "scaled signal in [EU]"=w134) -> ("error out"=w165:errorcluster, "scaled signal out [EU]"=w163:waveform(dbl))  [unwired: 8 in]
      n16 = Build Array (concatenate)(w134, w106) -> (w128:waveform(dbl)[])
      n17 = Compound Arithmetic op=ADD(w108, invert w112) -> (w114:i32)
      n18 = call-poly <vilib>:"Ramp Pattern.vi"("start"=w113, "end"=w108, "samples"=w114) -> ("Ramp Pattern"=w111:dbl[])  [unwired: 7 in, 1 out]
      n19 = call-poly <vilib>:"SVL AC & DC Level.vi"("scaled signal [EU]"=w163, "window"=w167, "error in (no error)"=w165) -> ("AC signal [EU]"=w164:waveform(dbl), "error out"=w166:errorcluster)  [unwired: 11 in, 4 out]
      n20 = call-poly <vilib>:"SVT Gain.vi"("scaled signal [EU]"=w164, "error in (no error)"=w166, "desired units"=T8 {"gain units"=enum."dB", "detected fundamental amplitude units"=enum."EU peak"}, "amplitude [EU peak]"=w135, "expected fundamental frequency [Hz]"=w115) -> ("detected fundamental\nfrequency [Hz]"=w116:dbl, "detected fundamental\namplitude"=w117:dbl, "complex spectrum"=w110:T17, "gain"=w132:dbl, "error out"=w168:errorcluster)  [unwired: 9 in, 1 out]
      n21 = Multiply(x=w116, y=w111) -> (x*y=w149:dbl[])
      n22 = call-poly <vilib>:"SVT THD and Harmonic Components.vi"("complex spectrum"=w110, "maximum harmonic"=w112, "error in (no error)"=w168, "desired units"=T7 {"THD units"=enum."%", "harmonic component amplitude units"=enum."EU peak", "detected fundamental amplitude units"=enum."EU peak"}, "expected fundamental frequency [Hz]"=w116) -> ("complex spectrum"=w141:T17, "THD"=w121:dbl, "harmonic components"=w137:cluster{"frequency [Hz]":dbl, "amplitude":dbl}[], "error out"=w145:errorcluster)  [unwired: 7 in, 4 out]
      n23 = call-poly <vilib>:"SV Convert to Data Object.vi"("complex spectrum"=w110) -> ("Spectrum Data"=w133:refnum<class "Data.lvclass">)  [unwired: 17 in, 1 out]
      n24 = call-poly <vilib>:"SVFA Extract Tone Information.vi"("complex spectrum"=w110, "expected frequencies [Hz]"=w149, "advanced span [Hz]"=0.0) -> ("detected tones"=w151:T18)  [unwired: 13 in, 3 out]
      n25 = for {
        tunnel: w151 -> [w169] mode=indexing
        tunnel: [w170] -> w158 mode=indexing
        n26 = Unbundle By Name(w169) -> ("amplitude [EU pk]"=w170:dbl)
      }
      n27 = for {
        tunnel: w137 -> [w172] mode=indexing
        tunnel: [w171] -> w160 mode=indexing
        n28 = Unbundle By Name(w172) -> ("amplitude"=w171:dbl)
      }
      n29 = call-poly <vilib>:"SVT SNR without Harmonics.vi"("complex spectrum"=w141, "frequency range"=w109, "maximum harmonic"=w112, "error in (no error)"=w145, "desired units"=T6 {"SNR units"=enum."dB", "detected fundamental amplitude units"=enum."EU rms"}, "expected fundamental frequency [Hz]"=w116) -> ("complex spectrum"=w143:T17, "SNR (without harmonics)"=w118:dbl, "SINAD"=w142:dbl, "THD"=w120:dbl, "error out"=w146:errorcluster)  [unwired: 6 in, 3 out]
      n30 = Negate(x=w142) -> (-x=w119:dbl)
      n31 = call-poly <vilib>:"SVT Dynamic Range.vi"("complex spectrum"=w143, "frequency range"=w109, "error in (no error)"=w146, "full scale amplitude [EU peak]"=w136, "expected fundamental\nfrequency [Hz]"=w116) -> ("dup complex spectrum"=w144:T17, "dynamic range"=w131:dbl, "error out"=w147:errorcluster)  [unwired: 9 in, 3 out]
      n32 = Square(x=w160) -> (x^2=w154:dbl[])
      n33 = Square(x=w117) -> (x^2=w157:dbl)
      n34 = Square(x=w158) -> (x^2=w152:dbl[])
      n35 = call-poly <vilib>:"SVT Spurious Free Dynamic Range.vi"("complex spectrum"=w144, "frequency range"=w109, "error in (no error)"=w147, "exclude harmonics"=TRUE, "expected fundamental\nfrequency [Hz]"=w116) -> ("spurious free dynamic range"=w130:dbl, "error out"=w129:errorcluster)  [unwired: 7 in, 6 out]
      n36 = Add Array Elements(numeric array=w154) -> (sum=w155:dbl)
      n37 = Add Array Elements(numeric array=w152) -> (sum=w161:dbl)
      n38 = Compound Arithmetic op=ADD(w155, w157, w161) -> (w156:dbl)
      n39 = Square Root(x=w156) -> (sqrt(x)=w159:dbl)
      n40 = Square Root(x=w161) -> (sqrt(x)=w153:dbl)
      n41 = Index Array(array=w160) -> (element #1=w122:dbl, element #2=w123:dbl, element #3=w124:dbl, element #4=w125:dbl, element #5=w126:dbl, element #6=w107:dbl)  [unwired: 6 in]
      n42 = Compound Arithmetic op=MULTIPLY(invert w159, w153, 100.0 ("y")) -> (w127:dbl)
    }
    frame #3 {
      # "Update Displays"
      "THD (dB)" <- w179
      "gain (dB)" <- w190
      "fundamental amplitude (V)" <- w176
      "fundamental frequency (Hz)" <- w174
      "2X amplitude (V)" <- w181
      "3X amplitude (V)" <- w182
      "4X amplitude (V)" <- w183
      "5X amplitude (V)" <- w184
      "6X amplitude (V)" <- w185
      "Spectrum with Cursors" <- w191
      "Waveforms with Cursors" <- w187
      "SNR (dB)" <- w177
      "THD (%)" <- w180
      "THD+N (dB)" <- w178
      "Dynamic Range (dB FS)" <- w189
      "SFDR (dB)" <- w188
      "Rub & Buzz distortion (%)" <- w186
      "7X amplitude (V)" <- w173
    }
    frame #4 {
      # "Report Errors"
      n43 = call <vilib>:"Simple Error Handler.vi"("error in (no error)"=w192) -> ()  [unwired: 4 in, 5 out]
    }
  }
